vi "Post_Process_Raw_data.vi"(0 "Select Plug Ins":bool, 2 "Post processed Results folder":path, 3 "No dialogs":bool, 5 "Save results to":T1(ring)=enum."Original Results Filenames", 7 "Add PP":bool=TRUE, 9 "Per Block Plug Ins Extra":string[](array[string]), 11 "Selected files":path[](array[path]), 12 "Current Results filenames":path[](array[path]), 13 "Results Plotter Channel names":string[](array[string]), 14 "Results Plotter Data":string[][](array[string])) -> (4 "Stopped":bool, 15 "Post processed Results folder Out":path)   [LabVIEW 2021]
uses:
  Anemometry Sub Vis/Controls/File_Selector_Type.ctl
  Anemometry Sub Vis/Controls/Setup.ctl
  Anemometry Sub Vis/Gen Trav/Multi_Run_Status.ctl
  Anemometry Sub Vis/Controls/Post_Process.ctl
  Anemometry Sub Vis/Controls/Save_Data.ctl
  Anemometry Sub Vis/Globals/Meas_global.vi
  Anemometry Sub Vis/Data_plotting_vis/Results_plotter_Global.vi
  Anemometry Sub Vis/Globals/Plug_in_data_global.vi
  Anemometry Sub Vis/Globals/Dynamic_call_global.ph.vi
panel:
  out "Time Taken (s)":dbl
  out "Single Filename":string
  out "nFiles not found":i32
  out "Files not Found":path[](array[path])
  out "Checking":i32
  in  "Previous Choice":path
  in  "Search String":string
  in  "Proceed?":bool
  in  "Pause Mode":enum16{"Continuous Running", "After Each File"}(ring)
  in  "At Dialog Prompt Post Process":T2=enum."All files listed in selected file"
  out "Files Processed":i32(slide) scale=0.0..20.0
  in  "stop":bool
  out "Files To Process":path[](array[path])
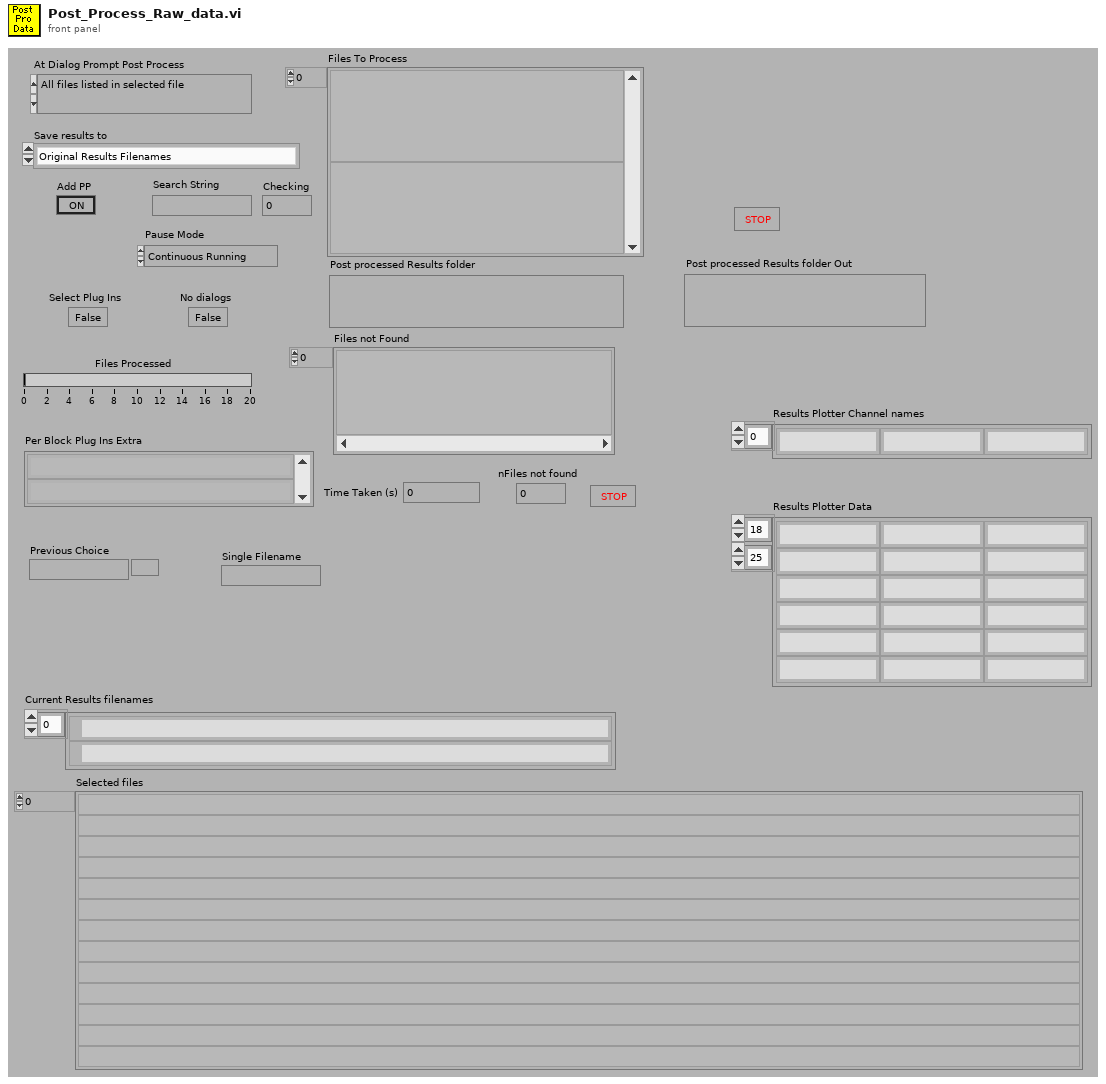
[diagram p1: front panel]
types:
  T1 = enum16{"A single file", "Original Results Filenames", "Current Results Filenames"}
  T2 = typedef "File_Selector_Type.ctl" = enum16{"The Selected File", "The Selected Folder", "Files containing the search string in the selected folder", "All files listed in selected file"}
  T3 = typedef "Setup.ctl" = enum16{"Run Program", "Show Setup", "Save Current Setup", "Setup Front Panel"}
  T4 = typedef "Multi_Run_Status.ctl" = enum16{"Continue", "Continue with Error", "Jump to Next Point", "Jump to Next Row", "Jump To Fall Back", "Terminate Run"}
  T5 = typedef "Save_Data.ctl" = enum16{"Save No Data", "Save Data"}
  T6 = typedef "Post_Process.ctl" = enum16{"Take New Data", "Post Process Raw Data File"}
  T7 = enum16{"Left Button", "Center Button", "Right Button", "Window Close"}
  T8 = typedef "Dispose_Channel.ctl" = enum16{"Always", "If Blank", "Never"}
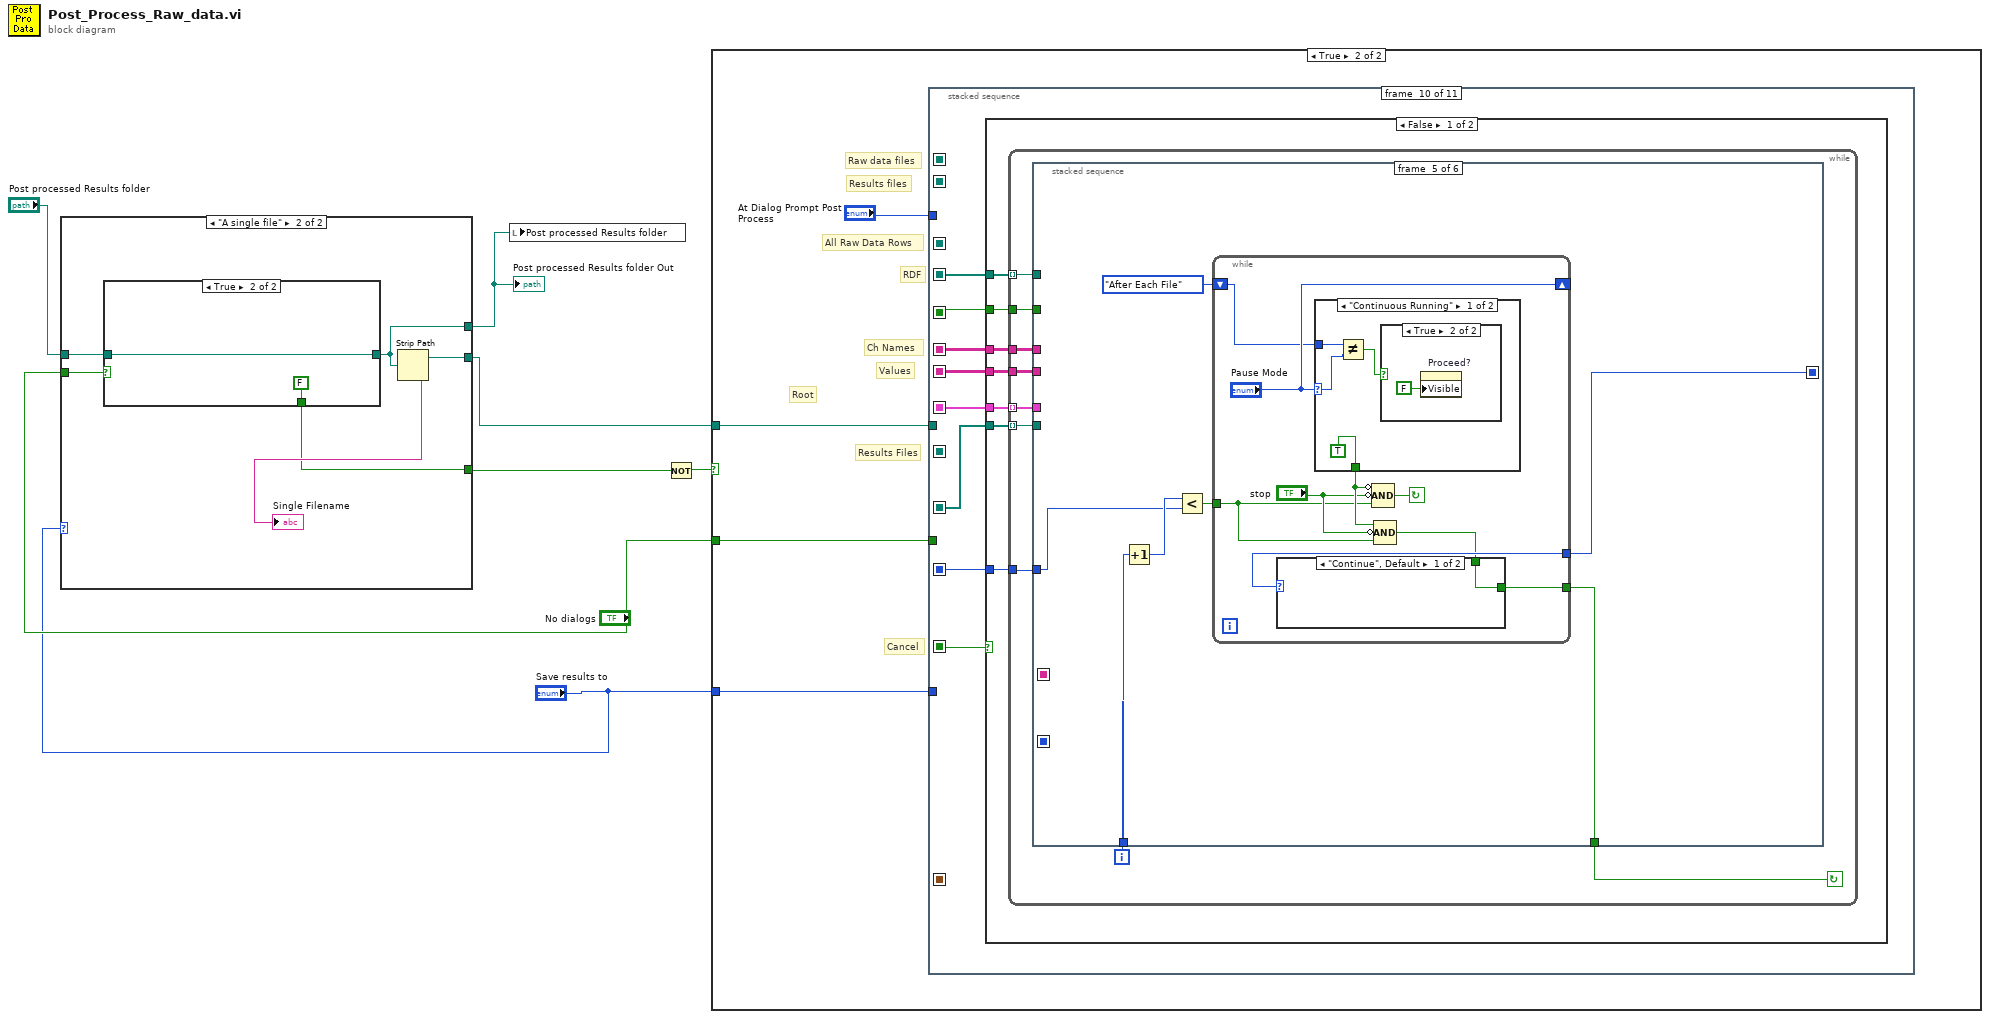
[diagram p0: block diagram]
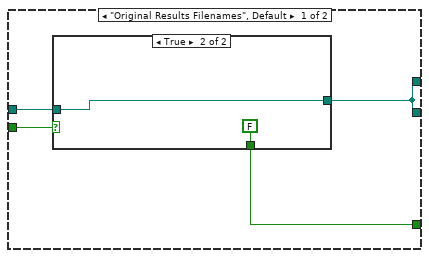
[diagram p2: hidden frame]
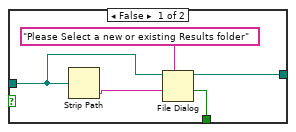
[diagram p3: hidden frame]
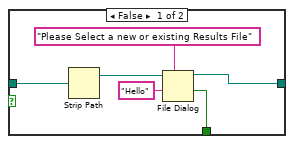
[diagram p4: hidden frame]
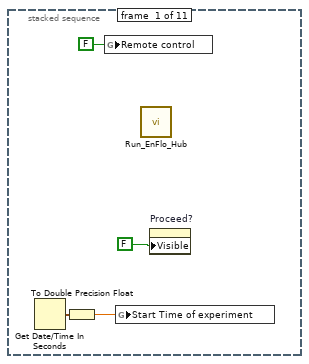
[diagram p6: hidden frame]
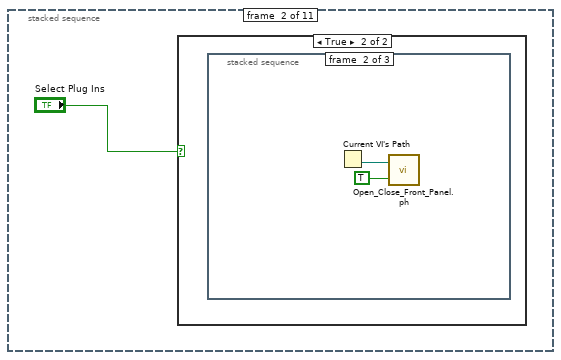
[diagram p7: hidden frame]
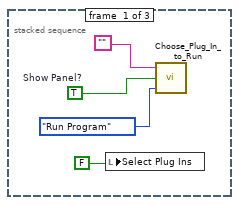
[diagram p9: hidden frame]
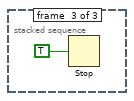
[diagram p10: hidden frame]
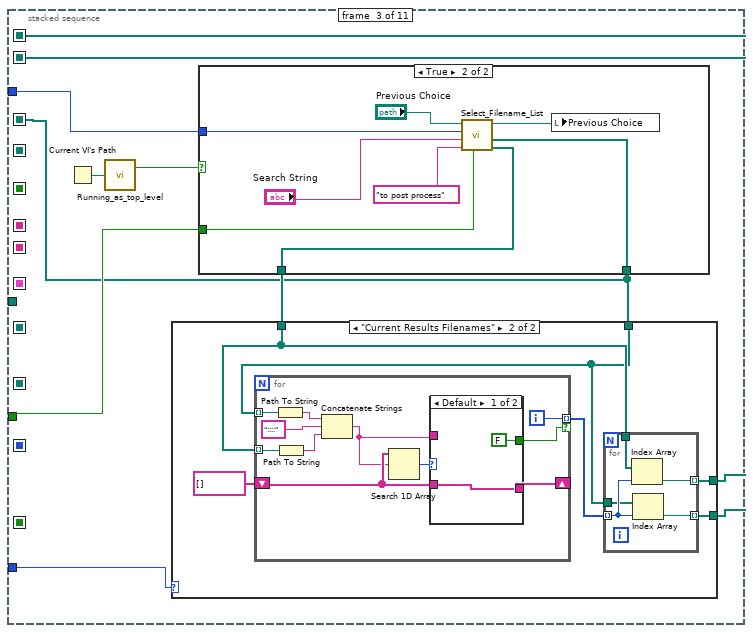
[diagram p11: hidden frame]
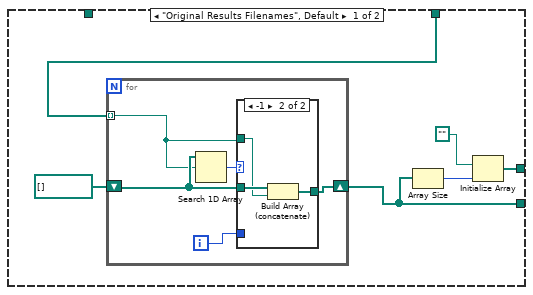
[diagram p12: hidden frame]
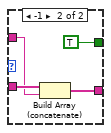
[diagram p14: hidden frame]
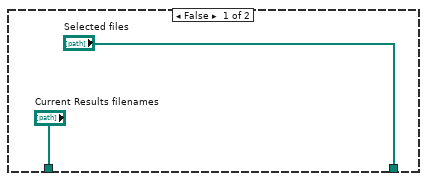
[diagram p15: hidden frame]
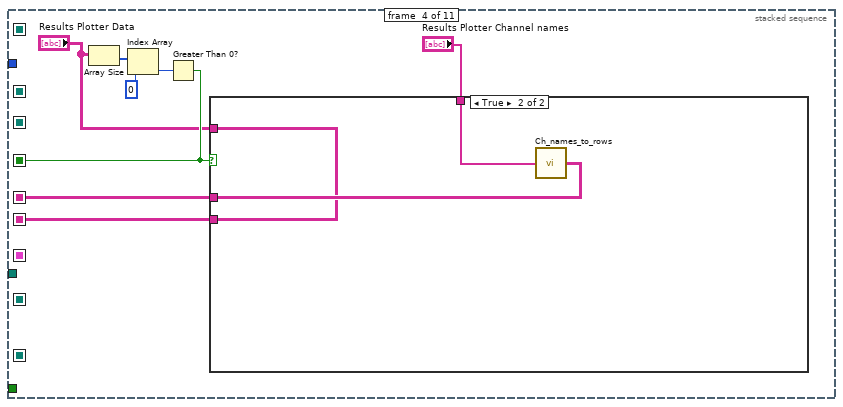
[diagram p16: hidden frame]
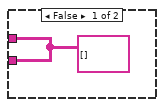
[diagram p17: hidden frame]
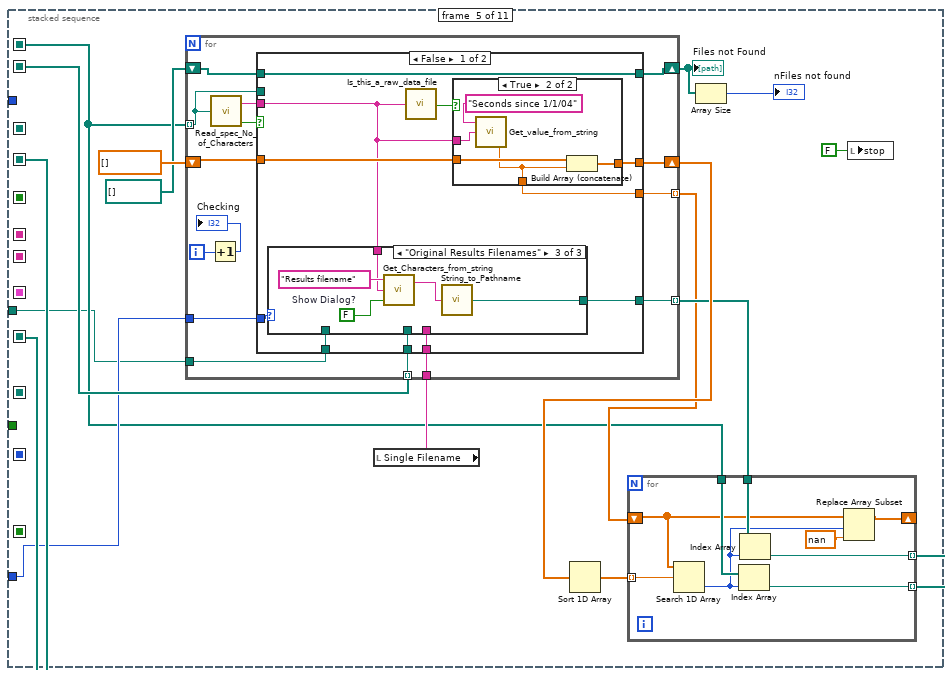
[diagram p18: hidden frame]
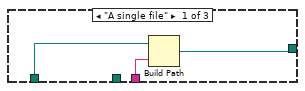
[diagram p19: hidden frame]
diagram:
  n1 = case shown="\"A single file\"" "Save results to" {
    tunnel: [w9 w21] -> w3
    tunnel: "Post processed Results folder" -> [w11 w24]
    tunnel: "No dialogs" -> [w10 w23]
    tunnel: [w9 w22] -> w7
    tunnel: [w8 w19] -> w2
    frame "Original Results Filenames", Default {
      n2 = case shown="True" w10 {
        tunnel: [w16 w18] -> w9
        tunnel: w11 -> [w13 w18]
        tunnel: [w12 FALSE ("cancelled")] -> w8
        frame False {
          n3 = Strip Path(path=w13) -> (name=w14:string)  [unwired: 1 out]
          n4 = File Dialog(7:"Please Select a new or existing Results folder" ("prompt"), 9:w14, 11:w13) -> (1:w12:bool, 3:w16:path)  [unwired: 1 in, 5 out]
        }
        frame True {
        }
      }
    }
    frame "A single file" {
      n5 = case shown="True" w23 {
        tunnel: w24 -> [w29 w32]
        tunnel: [w28 w32] -> w22
        tunnel: [w25 FALSE ("cancelled")] -> w19
        frame False {
          n6 = Strip Path(path=w29) -> (stripped path=w27:path)  [unwired: 1 out]
          n7 = File Dialog(7:"Please Select a new or existing Results File" ("prompt"), 9:"Hello" ("default name"), 11:w27) -> (1:w25:bool, 3:w28:path)  [unwired: 1 in, 5 out]
        }
        frame True {
        }
      }
      n8 = Strip Path(path=w22) -> (stripped path=w21:path, name=→"Single Filename":string)
    }
  }
  "Post processed Results folder Out" <- w7
  n9 = local write "Post processed Results folder"(w7) -> ()
  n10 = Not(x=w2) -> (.not. x?=w1:bool)
  n11 = case shown="True" w1 {
    tunnel: "Save results to" -> [_ w35]
    tunnel: "No dialogs" -> [_ w34]
    tunnel: w3 -> [_ w33]
    frame False {
    }
    frame True {
      # "RDF"
      # "All Raw Data Rows"
      # "Values"
      # "Ch Names"
      # "Cancel"
      # "Results files"
      # "Raw data files"
      # "Root"
      # "Results Files"
      n12 = stacked-sequence {
        seq-local: [_ _ _ _ w135 _ _ _ _ _ _] -> [_ _ _ _ _ _ _ w251 w261 w274 _]
        seq-local: [_ _ _ _ _ _ _ _ w266 _ _] -> [_ _ _ _ _ _ _ _ _ w273 _]
        seq-local: [_ _ w51 _ _ _ _ _ _ _ _] -> [_ _ _ _ w124 _ _ _ _ _ _]
        seq-local: [_ _ _ _ w133 _ _ _ _ _ _] -> [_ _ _ _ _ w200 _ _ _ _ _]
        seq-local: [_ _ _ _ _ w197 _ _ _ _ _] -> [_ _ _ _ _ _ w221 _ _ w272 w402]
        seq-local: [_ _ w52 _ _ _ _ _ _ _ _] -> [_ _ _ _ w129 _ _ _ _ _ _]
        seq-local: [_ _ _ w118 _ _ _ _ _ _ _] -> [_ _ _ _ _ _ _ _ _ w271 _]
        seq-local: [_ _ _ w117 _ _ _ _ _ _ _] -> [_ _ _ _ _ _ _ _ _ w269 _]
        seq-local: [_ _ _ w113 _ _ _ _ _ _ _] -> [_ _ _ _ _ _ _ _ _ w270 _]
        seq-local: [_ _ w49 _ _ _ _ _ _ _ _] -> [_ _ _ _ _ _ _ w250 _ _ _]
        seq-local: [_ _ _ _ _ _ w223 _ _ _ _] -> [_ _ _ _ _ _ _ _ _ w268 _]
        seq-local: [_ _ _ _ _ _ _ w249 _ _ _] -> [_ _ _ _ _ _ _ _ _ w267 _]
        seq-local: [_ _ _ _ _ _ _ _ w260 _ _] -> [_ _ _ _ _ _ _ _ _ _ w398]
        tunnel: "At Dialog Prompt Post Process" -> [_ _ w57 _ _ _ _ _ _ _ _]
        tunnel: w34 -> [_ _ w56 _ _ _ w224 _ _ _ _]
        tunnel: w35 -> [_ _ w50 _ w128 w199 _ _ _ _ _]
        tunnel: w33 -> [_ _ _ _ w123 w196 _ _ _ _ _]
        frame #0 {
          n13 = Get Date/Time In Seconds() -> (seconds since 1Jan1904=w37:timestamp)
          n14 = To Double Precision Float(number=w37) -> (double precision float=w38:dbl)
          n15 = global write "Meas_global.vi" "Remote control"(FALSE ("Remote control")) -> ()
          n16 = global write "Meas_global.vi" "Start Time of experiment"(w38) -> ()
          n17 = call "Run_EnFlo_Hub.vi"() -> ()  [unwired: 1 in, 7 out]
          n18 = property on="Proceed?" class="Bool"("Visible"=FALSE ("Write Attribute")) -> ()  [unwired: 2 in, 2 out]
        }
        frame #1 {
          n19 = case shown="True" "Select Plug Ins" {
            frame False {
            }
            frame True {
              n20 = stacked-sequence {
                frame #0 {
                  w45 = TRUE  # Show Panel?
                  n21 = local write "Select Plug Ins"(FALSE ("Select Local ADAM Channels")) -> ()
                  n22 = call "Choose_Plug_In_to_Run.vi"("setup"=Setup."Run Program", "Show Panel?"=w45, "Setup String In"="") -> ()  [unwired: 2 out]
                }
                frame #1 {
                  n23 = Current VI's Path() -> (path=w47:path)
                  n24 = call "Open_Close_Front_Panel.ph.vi"("openWindow (T)"=TRUE ("Front Panel Window:Open"), "VI path"=w47) -> ()  [unwired: 1 in, 1 out]
                }
                frame #2 {
                  n25 = Stop(stop? (T)=TRUE) -> ()
                }
              }
            }
          }
        }
        frame #2 {
          n26 = Current VI's Path() -> (path=w55:path)
          n27 = call "Running_as_top_level.vi"("Vi path name"=w55) -> ("Top Level"=w54:bool)  [unwired: 1 out]
          n28 = case shown="True" w54 {
            tunnel: w57 -> [_ w110]
            tunnel: w56 -> [_ w105]
            tunnel: ["Selected files" w104] -> w49
            tunnel: ["Current Results filenames" w103] -> w53
            frame False {
            }
            frame True {
              n29 = call "Select_Filename_List.vi"("No dialogs"=w105, "File Type"="to post process", "Search String"="Search String", "At Dialog Prompt Post Process"=w110, "Previous Choice"="Previous Choice") -> ("Current Results filenames"=w103:path[], "Selected files"=w104:path[], "Choosen path"=w106:path)  [unwired: 1 out]
              n30 = local write "Previous Choice"(w106) -> ()
            }
          }
          n31 = case shown="\"Current Results Filenames\"" w50 {
            tunnel: w49 -> [w63 w76]
            tunnel: w53 -> [_ w77]
            tunnel: [w59 w75] -> w52
            tunnel: [w61 w74] -> w51
            frame "Original Results Filenames", Default {
              n32 = for {
                shift-right: [w67] -> w61
                shift-left: path[] [] -> [w68]
                tunnel: w63 -> [w64] mode=indexing
                i -> [w65]
                n33 = Search 1D Array(1D array=w68, element=w64) -> (index of element=w66:i32)  [unwired: 1 out]
                n34 = case shown="-1" w66 {
                  tunnel: w68 -> [w69 w72]
                  tunnel: [w69 w71] -> w67
                  tunnel: w64 -> [_ w70]
                  tunnel: w65 -> [_ _]
                  frame 0, Default {
                  }
                  frame -1 {
                    n35 = Build Array (concatenate)(w72, w70) -> (w71:path[])
                  }
                }
              }
              n36 = Array Size(array=w61) -> (size(s)=w60:i32)
              n37 = Initialize Array(path "", w60) -> (w59:path[])
            }
            frame "Current Results Filenames" {
              n38 = for {
                shift-right: [w93] -> _
                shift-left: string[] [] -> [w94]
                tunnel: w76 -> [w92] mode=indexing
                tunnel: w77 -> [w89] mode=indexing
                tunnel: [w85] -> w73 mode=indexing if=w84
                i -> [w85]
                n39 = Path To String(path=w92) -> (string=w91:string)
                n40 = Path To String(path=w89) -> (string=w88:string)
                n41 = Concatenate Strings(w91, "::::" ("string"), w88) -> (w87:string)
                n42 = Search 1D Array(1D array=w94, element=w87) -> (index of element=w86:i32)  [unwired: 1 out]
                n43 = case shown="Default" w86 {
                  tunnel: w94 -> [w96 w100]
                  tunnel: [w96 w99] -> w93
                  tunnel: w87 -> [_ w98]
                  tunnel: [FALSE TRUE] -> w84
                  frame Default {
                  }
                  frame -1 {
                    n44 = Build Array (concatenate)(w100, w98) -> (w99:string[])
                  }
                }
              }
              n45 = for {
                tunnel: w73 -> [w83] mode=indexing
                tunnel: w77 -> [w82]
                tunnel: w76 -> [w81]
                tunnel: [w80] -> w75 mode=indexing
                tunnel: [w79] -> w74 mode=indexing
                n46 = Index Array(array=w82, index=w83) -> (element=w80:path)
                n47 = Index Array(array=w81, index=w83) -> (element=w79:path)
              }
            }
          }
        }
        frame #3 {
          n48 = Array Size(array="Results Plotter Data") -> (size(s)=w116:i32[])
          n49 = Index Array(array=w116, index=0) -> (element=w114:i32)
          n50 = Greater Than 0?(x=w114) -> (x > 0?=w113:bool)
          n51 = case shown="True" w113 {
            tunnel: [w119 w122] -> w118
            tunnel: [w119 w120] -> w117
            tunnel: "Results Plotter Data" -> [_ w120]
            tunnel: "Results Plotter Channel names" -> [_ w121]
            frame False {
              w119 = string[][] [] ("3 Row names")
            }
            frame True {
              n52 = call "Ch_names_to_rows.vi"("Channel Names"=w121) -> ("3 Row names"=w122:string[][])
            }
          }
        }
        frame #4 {
          n53 = local read "Single Filename"() -> (w127:string)
          n54 = for {
            tunnel: w124 -> [w157] mode=indexing
            shift-right: [w161] -> w138
            shift-left: dbl[] [] -> [w162]
            shift-right: [w158] -> w131
            shift-left: path[] [] -> [w159]
            tunnel: w129 -> [w154] mode=indexing
            tunnel: w128 -> [w153]
            tunnel: w123 -> [w152]
            tunnel: w127 -> [w151]
            tunnel: [w150] -> w126 mode=indexing
            tunnel: [w149] -> w125 mode=indexing
            i -> [w160]
            n55 = Increment(x=w160) -> (x+1=→"Checking":i32)
            n56 = call "Read_spec_No_of_Characters.vi"("Filename"=w157) -> ("character string"=w156:string, "Error?"=w155:bool)
            n57 = case shown="False" w155 {
              tunnel: w162 -> [w173 w195]
              tunnel: [w172 w195] -> w161
              tunnel: w157 -> [_ w193]
              tunnel: w159 -> [w170 w194]
              tunnel: [w170 w192] -> w158
              tunnel: w156 -> [w169 _]
              tunnel: w154 -> [w167 w191]
              tunnel: w153 -> [w168 _]
              tunnel: w152 -> [w166 _]
              tunnel: w151 -> [w165 _]
              tunnel: [w164 w191] -> w150
              tunnel: [w163 0.0 ("Value")] -> w149
              frame False {
                n58 = case shown="\"Original Results Filenames\"" w168 {
                  tunnel: [w176 w177 w180] -> w164
                  tunnel: w169 -> [_ _ w178]
                  tunnel: w167 -> [_ w177 _]
                  tunnel: w166 -> [w175 _ _]
                  tunnel: w165 -> [w174 _ _]
                  frame "A single file" {
                    n59 = Build Path(base path=w175, name or relative path=w174) -> (appended path=w176:path)
                  }
                  frame "Current Results Filenames" {
                  }
                  frame "Original Results Filenames" {
                    w181 = FALSE  # Show Dialog?
                    n60 = call "Get_Characters_from_string.vi"("Show Dialog?"=w181, "Input string"=w178, "Variable name"="Results filename") -> ("Value"=w179:string)  [unwired: 1 out]
                    n61 = call "String_to_Pathname.vi"("Input String"=w179) -> ("path"=w180:path)
                  }
                }
                n62 = call "Is_this_a_raw_data_file.vi"("character string"=w169) -> ("Raw Dat File?"=w171:bool)  [unwired: 2 out]
                n63 = case shown="True" w171 {
                  tunnel: w173 -> [w184 w186]
                  tunnel: [w184 w189] -> w172
                  tunnel: w169 -> [_ w187]
                  tunnel: [0.0 ("Value") w185] -> w163
                  frame False {
                  }
                  frame True {
                    n64 = call "Get_value_from_string.vi"("Input string"=w187, "Variable name"="Seconds since 1/1/04") -> ("Value"=w185:dbl)  [unwired: 1 in, 1 out]
                    n65 = Build Array (concatenate)(w186, w185) -> (w189:dbl[])
                  }
                }
              }
              frame True {
                n66 = Build Array (concatenate)(w194, w193) -> (w192:path[])
              }
            }
          }
          "Files not Found" <- w131
          n67 = Sort 1D Array(array=w138) -> (sorted array=w137:dbl[])
          n68 = for {
            tunnel: w137 -> [w147] mode=indexing
            tunnel: w124 -> [w146]
            tunnel: [w145] -> w135 mode=indexing
            tunnel: w126 -> [w144]
            tunnel: [w143] -> w133 mode=indexing
            shift-right: [w142] -> _
            shift-left: w125 -> [w139]
            n69 = Search 1D Array(1D array=w139, element=w147) -> (index of element=w141:i32)  [unwired: 1 out]
            n70 = Index Array(array=w146, index=w141) -> (element=w145:path)
            n71 = Index Array(array=w144, index=w141) -> (element=w143:path)
            n72 = Replace Array Subset(array=w139, new element=nan ("new element/subarray"), index=w141) -> (w142:dbl[])
          }
          n73 = Array Size(array=w131) -> (size(s)=→"nFiles not found":i32)
          n74 = local write "stop"(FALSE ("stop")) -> ()
        }
        frame #5 {
          n75 = case shown="\"Original Results Filenames\"" w199 {
            tunnel: [FALSE "Add PP"] -> w198
            tunnel: w199 -> [_ _]
            frame "A single file", Default {
            }
            frame "Original Results Filenames" {
            }
          }
          n76 = for {
            tunnel: w200 -> [w215] mode=indexing
            tunnel: w198 -> [w210]
            tunnel: w196 -> [w209]
            tunnel: [w207] -> w197 mode=indexing
            n77 = Strip Path(path=w215) -> (name=w206:string)  [unwired: 1 out]
            n78 = call "Remove illegal characters fr filename.vi"("Filename In"=w206) -> ("Cleaned Filename"=w205:string)  [unwired: 2 in]
            n79 = call "Add_filename_suffix.vi"("Filename"=w205) -> ("Original Suffix"=w213:string, "Base name"=w204:string)  [unwired: 1 in, 2 out]
            n80 = case shown="False" w210 {
              tunnel: [w216 w218] -> w203
              tunnel: w204 -> [w216 w217]
              frame False {
              }
              frame True {
                n81 = Concatenate Strings(w217, "_pp" ("Substring")) -> (w218:string)
              }
            }
            n82 = Empty String/Path?(string/path=w213) -> (empty?=w214:bool)
            n83 = Select(t=".xls", s=w214, f=w213) -> (s? t:f=w212:string)
            n84 = Concatenate Strings(w203, w212) -> (w208:string)
            n85 = Build Path(base path=w209, name or relative path=w208) -> (appended path=w207:path)
          }
        }
        frame #6 {
          n86 = Path To String(path=w221) -> (string=w222:string[])
          n87 = call "Analyse_string_array.vi"("String array"=w222) -> ("Unique strings"=w220:string[])  [unwired: 2 out]
          n88 = case shown="False" w224 {
            tunnel: [w226 FALSE ("stop? (T)")] -> w223
            tunnel: w220 -> [w225 w245]
            frame False {
              n89 = for {
                tunnel: w225 -> [w229] mode=indexing
                tunnel: [w228] -> w226
                stop <- w228 stop-if-true
                n90 = String To Path(string=w229) -> (path=w227:path)
                n91 = call "Create_directory_path.vi"("Path name"=w227) -> ()  [unwired: 2 in, 2 out]
                n92 = call "Does_file_exist_(simple).vi"("Pathname"=w227) -> ("exists?"=w230:bool)
                n93 = case shown="True" w230 {
                  tunnel: w227 -> [_ w235]
                  tunnel: [FALSE ("stop? (T)") w234] -> w228
                  frame False {
                  }
                  frame True {
                    n94 = Format Into String(format string="%s\nAlready exists. ", w235) -> (resulting string=w238:string)  [unwired: 2 in, 1 out]
                    n95 = call <vilib>:"Three Button Dialog.vi"("Allow user to close window? (TRUE)"=FALSE, "Center Button Text (\"No\")"="Append" ("Center Button Text (\"No\")"), "Left Button Text (\"Yes\")"="Overwrite" ("Left Button Text (\"Yes\")"), "message"=w238) -> ("Which Button?"=w236:T7)  [unwired: 7 in]
                    n96 = case shown="\"Center Button\"" w236 {
                      tunnel: w235 -> [w241 _ _ _]
                      tunnel: [FALSE ("stop? (T)") FALSE ("stop? (T)") TRUE ("stop? (T)") FALSE ("stop? (T)")] -> w234
                      frame "Left Button" {
                        n97 = Delete(path (use dialog)=w241) -> ()  [unwired: 4 in, 3 out]
                      }
                      frame "Center Button" {
                      }
                      frame "Right Button" {
                      }
                      frame "Window Close" {
                      }
                    }
                  }
                }
              }
            }
            frame True {
              n98 = for {
                tunnel: w245 -> [w248] mode=indexing
                n99 = String To Path(string=w248) -> (path=w247:path)
                n100 = call "Create_directory_path.vi"("Path name"=w247) -> ()  [unwired: 2 in, 2 out]
              }
            }
          }
        }
        frame #7 {
          n101 = for {
            tunnel: w251 -> [w255] mode=indexing
            tunnel: w250 -> [w254]
            tunnel: [w252] -> w249 mode=indexing
            n102 = for {
              tunnel: w255 -> [w259]
              tunnel: w254 -> [w258] mode=indexing
              tunnel: [w257] -> w253 mode=indexing if=w256
              i -> [w257]
              n103 = Equal?(x=w259, y=w258) -> (x = y?=w256:bool)
            }
            n104 = Bundle(w253) -> (w252:cluster{i32[]})  [unwired: 1 in]
          }
        }
        frame #8 {
          w262 = 0 ("Files Processed")
          n105 = Get Date/Time In Seconds() -> (seconds since 1Jan1904=w260:timestamp)
          n106 = Array Size(array=w261) -> (size(s)=w266:i32)
          n107 = Array Size(array=w261) -> (size(s)=w264:i32)
          n108 = Build Array(w262) -> (w263:i32[])
          n109 = property on="Files Processed" class="Slide (strict)"("Scale.Range:Minimum"=0.0 ("Write Attribute"), "Scale.Range:Maximum"=w264) -> ()  [unwired: 2 in, 2 out]
          n110 = property on="Attribute Node" class="Arr (strict)"("Index Values"=w263) -> ()  [unwired: 2 in, 2 out]
          n111 = local write "Files Processed"(w262) -> ()
          "Files To Process" <- w261
        }
        frame #9 {
          n112 = case shown="False" w268 {
            tunnel: w274 -> [w281 _]
            tunnel: w273 -> [w280 _]
            tunnel: w272 -> [w279 _]
            tunnel: w271 -> [w278 _]
            tunnel: w270 -> [w277 _]
            tunnel: w269 -> [w276 _]
            tunnel: w267 -> [w275 _]
            frame False {
              n113 = while {
                tunnel: w279 -> [w286] mode=indexing
                tunnel: w280 -> [w289]
                tunnel: w281 -> [w290] mode=indexing
                tunnel: w278 -> [w285]
                tunnel: w277 -> [w284]
                tunnel: w276 -> [w283]
                tunnel: w275 -> [w282] mode=indexing
                i -> [w288]
                stop <- w287 continue-if-true
                n114 = stacked-sequence {
                  seq-local: [_ _ _ w355 _ _] -> [_ _ _ _ w369 _]
                  seq-local: [w295 _ _ _ _ _] -> [_ w313 _ _ _ _]
                  seq-local: [w291 _ _ _ _ _] -> [_ w312 _ _ _ _]
                  tunnel: w286 -> [_ _ _ w356 _ _]
                  tunnel: w290 -> [_ _ _ w354 _ _]
                  tunnel: w289 -> [_ _ _ _ w371 _]
                  tunnel: w288 -> [_ _ _ _ w370 w395]
                  tunnel: [_ _ _ _ w368 _] -> w287
                  tunnel: w285 -> [_ w317 _ _ _ _]
                  tunnel: w284 -> [_ w316 _ _ _ _]
                  tunnel: w283 -> [w293 _ _ _ _ _]
                  tunnel: w282 -> [w292 _ _ _ _ _]
                  frame #0 {
                    n115 = Unbundle(w292) -> (w294:i32[])
                    n116 = for {
                      tunnel: w293 -> [w299]
                      tunnel: [w298] -> w291 mode=indexing
                      tunnel: w294 -> [w297] mode=indexing
                      n117 = Index Array(array=w299, index (row)=w297) -> (element=w298:string[])  [unwired: 1 in]
                    }
                    n118 = global read "Results_plotter_Global.vi" "Dispose"() -> (w296:T8[])
                    n119 = for {
                      tunnel: w296 -> [w303] mode=indexing
                      tunnel: [w300] -> w295 mode=indexing if=w302
                      tunnel: w291 -> [w301]
                      i -> [w300]
                      n120 = case shown="\"If Blank\"" w303 {
                        tunnel: [FALSE TRUE w309] -> w302
                        tunnel: w301 -> [_ _ w311]
                        tunnel: w300 -> [_ _ w308]
                        frame "Always" {
                        }
                        frame "Never" {
                        }
                        frame "If Blank" {
                          n121 = Index Array(array=w311, index (row)=w308) -> (element=w307:string[])  [unwired: 1 in]
                          n122 = Concatenate Strings(w307) -> (w306:string)
                          n123 = Empty String/Path?(string/path=w306) -> (empty?=w310:bool)
                          n124 = Not(x=w310) -> (.not. x?=w309:bool)
                        }
                      }
                    }
                  }
                  frame #1 {
                    n125 = case shown="True" w316 {
                      tunnel: w317 -> [_ w325]
                      tunnel: w312 -> [_ w323]
                      tunnel: [w318 w320] -> w315
                      tunnel: [w318 w323] -> w314
                      tunnel: w313 -> [_ w324]
                      frame False {
                        w318 = string[][] [] ("3 Row names")
                      }
                      frame True {
                        n126 = global read "Results_plotter_Global.vi" "Precision"() -> (w319:string[])
                        n127 = for {
                          tunnel: w324 -> [w329]
                          tunnel: w323 -> [w328] mode=indexing
                          tunnel: w319 -> [w327]
                          tunnel: [w326] -> w322 mode=indexing
                          n128 = for {
                            tunnel: w329 -> [w339] mode=indexing
                            tunnel: w328 -> [w341]
                            tunnel: w327 -> [w340]
                            tunnel: [w333] -> w326 mode=indexing
                            n129 = Index Array(array=w341, index=w339) -> (element=w332:string)
                            n130 = Index Array(array=w340, index=w339) -> (element=w331:string)
                            n131 = Fract/Exp String To Number(string=w332) -> (offset past number=w337:i32, number=w334:dbl)  [unwired: 3 out]
                            n132 = String Length(string=w332) -> (length=w338:i32)
                            n133 = Equal?(x=w338, y=w337) -> (x = y?=w335:bool)
                            n134 = Empty String/Path?(string/path=w332) -> (empty?=w336:bool)
                            n135 = Compound Arithmetic op=AND(invert w336, w335) -> (w330:bool)
                            n136 = case shown="False" w330 {
                              tunnel: w331 -> [_ w344]
                              tunnel: w334 -> [_ w345]
                              tunnel: [w342 w343] -> w333
                              tunnel: w332 -> [w342 _]
                              frame False {
                              }
                              frame True {
                                n137 = call "Number_2_string.vi"("precision"=w344, "number"=w345) -> ("String"=w343:string)
                              }
                            }
                          }
                        }
                        n138 = for {
                          tunnel: w324 -> [w347]
                          tunnel: w325 -> [w348] mode=indexing
                          tunnel: [w346] -> w321 mode=indexing
                          n139 = for {
                            tunnel: w347 -> [w351] mode=indexing
                            tunnel: w348 -> [w350]
                            tunnel: [w349] -> w346 mode=indexing
                            n140 = Index Array(array=w350, index=w351) -> (element=w349:string)
                          }
                        }
                        n141 = Build Array (concatenate)(w321, w322) -> (w320:string[][])
                      }
                    }
                    n142 = global write "Plug_in_data_global.vi" "Results File Plotter Rows"(w314) -> ()
                    n143 = global write "Plug_in_data_global.vi" "Templated Results header"(w315) -> ()
                  }
                  frame #2 {
                    n144 = global write "Dynamic_call_global.ph.vi" "Per Block Plug Ins Extra"("Per Block Plug Ins Extra") -> ()
                  }
                  frame #3 {
                    n145 = call "Does_file_exist_(simple).vi"("Pathname"=w354) -> ("exists?"=w353:bool)
                    n146 = call "Program_Active.vi"() -> ()  [unwired: 1 in]
                    n147 = case shown="True" w353 {
                      tunnel: w356 -> [_ w366]
                      tunnel: w354 -> [w358 w365]
                      tunnel: [Multi_Run_Status."Continue" ("Status Out") w364] -> w355
                      frame False {
                        n148 = local read "Files not Found"() -> (w360:path[])
                        n149 = Build Array (concatenate)(w360, w358) -> (w359:path[])
                        n150 = local write "Files not Found"(w359) -> ()
                      }
                      frame True {
                        n151 = call "Measurement.vi"("setup"=Setup."Run Program", "Post Process"=Post_Process."Post Process Raw Data File", "File"=Save_Data."Save Data", "Results file"=w366, "Raw data file"=w365) -> ("Status Out"=w364:T4)  [unwired: 1 in, 13 out]
                      }
                    }
                  }
                  frame #4 {
                    n152 = Increment(x=w370) -> (x+1=w373:i32)
                    n153 = Less?(x=w373, y=w371) -> (x < y?=w372:bool)
                    n154 = while {
                      tunnel: [w381] -> w368
                      tunnel: w369 -> [w382]
                      tunnel: w372 -> [w377]
                      shift-right: ["Pause Mode"] -> _
                      shift-left: enum16{"Continuous Running", "After Each File"}."After Each File" ("Pause Mode") -> [w374]
                      stop <- w380 continue-if-true
                      n155 = case shown="\"Continuous Running\"" "Pause Mode" {
                        selector: "Pause Mode" -> [w384 _]
                        tunnel: [TRUE "Proceed?"] -> w379
                        tunnel: w374 -> [w385 _]
                        frame "Continuous Running" {
                          n156 = Not Equal?(x=w385, y=w384) -> (x != y?=w383:bool)
                          n157 = case shown="True" w383 {
                            frame False {
                            }
                            frame True {
                              n158 = property on="Proceed?" class="Bool"("Visible"=FALSE) -> ()  [unwired: 2 in, 2 out]
                            }
                          }
                        }
                        frame "After Each File" {
                          w389 = TRUE ("Blinking")
                          n159 = Wait (ms)(milliseconds to wait=u32 100 ("f")) -> ()  [unwired: 1 out]
                          n160 = property on="Proceed?" class="Bool"("Visible"=w389, "Key Focus"=w389, "Blinking"=w389) -> ()  [unwired: 2 in, 2 out]
                        }
                      }
                      n161 = Compound Arithmetic op=AND(invert w379, invert "stop", w377) -> (w380:bool)
                      n162 = Compound Arithmetic op=AND(w379, invert "stop", w377) -> (w376:bool)
                      n163 = case shown="\"Continue\", Default" w382 {
                        tunnel: [w391 FALSE] -> w381
                        tunnel: w376 -> [w391 _]
                        frame "Continue", Default {
                        }
                        frame "Terminate Run" {
                        }
                      }
                    }
                  }
                  frame #5 {
                    w393 = string[][] [] ("Results File Plotter Rows")
                    n164 = Increment(x=w395) -> (x+1=w394:i32)
                    "Files Processed" <- w394
                    n165 = global write "Plug_in_data_global.vi" "Templated Results header"(w393) -> ()
                    n166 = Build Array(w394) -> (w396:i32[])
                    n167 = global write "Plug_in_data_global.vi" "Results File Plotter Rows"(w393) -> ()
                    n168 = property on="Attribute Node" class="Arr (strict)"("Index Values"=w396) -> ()  [unwired: 2 in, 2 out]
                  }
                }
              }
            }
            frame True {
            }
          }
        }
        frame #10 {
          n169 = Get Date/Time In Seconds() -> (seconds since 1Jan1904=w399:timestamp)
          n170 = Subtract(x=w399, y=w398) -> (x-y=→"Time Taken (s)":dbl)
          n171 = Path To String(path=w402) -> (string=w404:string[])
          n172 = call "Analyse_string_array.vi"("String array"=w404) -> ("Unique strings"=w403:string[])  [unwired: 2 out]
          n173 = String To Path(string=w403) -> (path=w401:path[])
          n174 = for {
            tunnel: w401 -> [w408] mode=indexing
            w409 = FALSE  # Lock File
            n175 = call "Lock_File.vi"("Lock File"=w409, "path"=w408) -> ()  [unwired: 1 in, 3 out]
          }
          n176 = local read "stop"() -> (→"Stopped":bool)
          n177 = Build Array(0) -> (w406:i32[])
          n178 = property on="Attribute Node" class="Arr (strict)"("Index Values"=w406) -> ()  [unwired: 2 in, 2 out]
          n179 = property on="Proceed?" class="Bool"("Visible"=FALSE ("Write Attribute")) -> ()  [unwired: 2 in, 2 out]
        }
      }
    }
  }
